vi "ALARM Catch Error.vi"(8 "error in (no error)":errorcluster, 9 "Data":variant, 10 "Message Queues out":T2, 11 "Hardware Resources in":T1={"LOG REF"=refnum, "Writer Queue"=refnum, "Log Path"=path "", "UPS standby"=FALSE, "status code"=5001, "SP"=[], "Over Sens Status"=[]}) -> (0 "error out":errorcluster, 3 "Hardware Resources out":T1={"LOG REF"=refnum, "Writer Queue"=refnum, "Log Path"=path "", "UPS standby"=FALSE, "status code"=5001, "SP"=[], "Over Sens Status"=[]})   [LabVIEW 2020, in "QCT ALARM.lvlib"]
uses:
  QCT ALARM.lvlib
  support/Message Queue/All Message Queues.ctl
  support/Message Queue/Message Cluster.ctl
  ALARM Configuration.ctl
  support/HW Message Cluster.ctl
  support/Message Queue/Enqueue Message (Single).vi
  support/Message Queue/Message Queue.lvlib
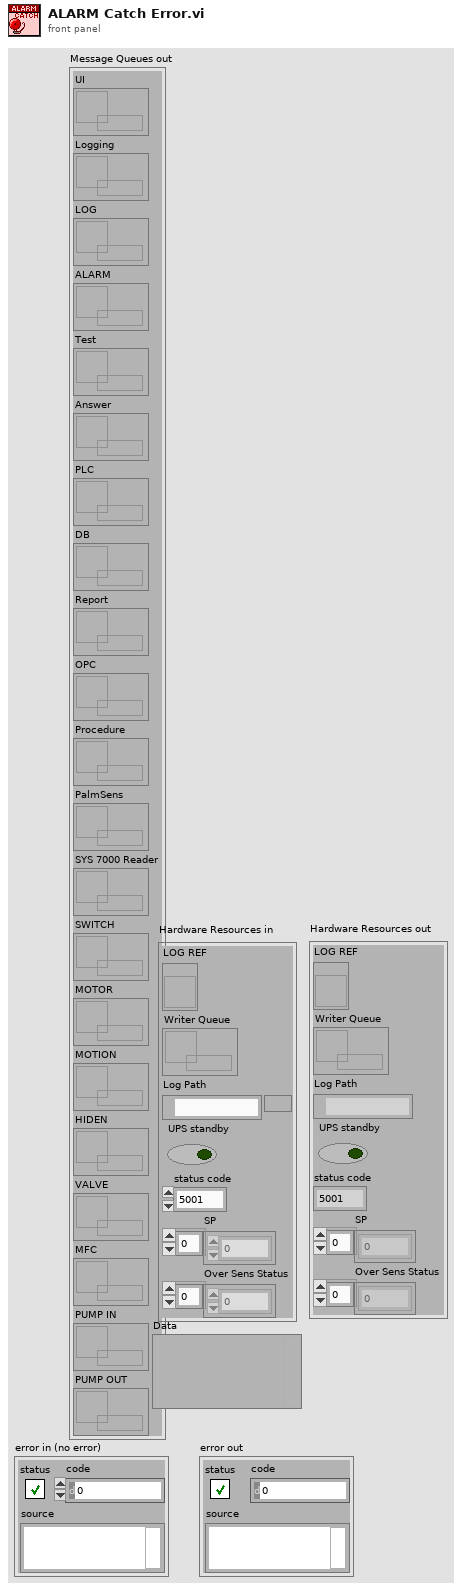
[diagram p1: front panel]
types:
  T1 = typedef "QCT ALARM.lvlib/ALARM Configuration.ctl" = cluster{"LOG REF":refnum<vi>, "Writer Queue":refnum<queue>, "Log Path":path, "UPS standby":bool, "status code":i32, "SP":dbl[], "Over Sens Status":dbl[]}
  T2 = typedef "Message Queue.lvlib/All Message Queues.ctl" = cluster{"UI":refnum<queue>, "Logging":refnum<queue>, "LOG":refnum<queue>, "ALARM":refnum<queue>, "Test":refnum<queue>, "Answer":refnum<queue>, "PLC":refnum<queue>, "DB":refnum<queue>, "Report":refnum<queue>, "OPC":refnum<queue>, "Procedure":refnum<queue>, "PalmSens":refnum<queue>, "SYS 7000 Reader":refnum<queue>, "SWITCH":refnum<queue>, "MOTOR":refnum<queue>, "MOTION":refnum<queue>, "HIDEN":refnum<queue>, "VALVE":refnum<queue>, "MFC":refnum<queue>, "PUMP IN":refnum<queue>, "PUMP OUT":refnum<queue>}
  T3 = typedef "Message Queue.lvlib/Message Cluster.ctl" = cluster{"Message":string, "Message Data":variant}
  T4 = typedef "Message Queue.lvlib/HW Message Cluster.ctl" = cluster{"Writer Queue":refnum<queue>, "Writer Data":T3}
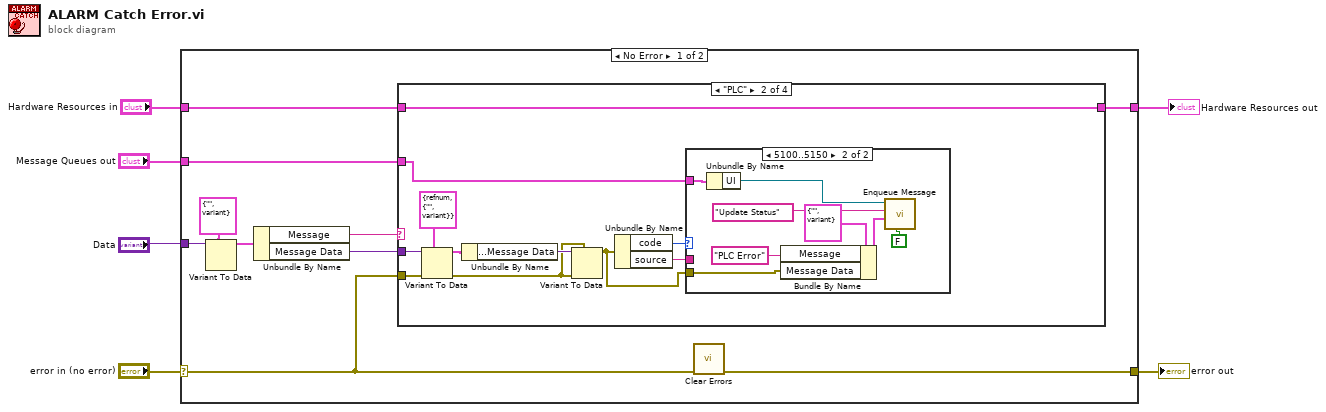
[diagram p0: block diagram]
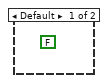
[diagram p3: hidden frame]
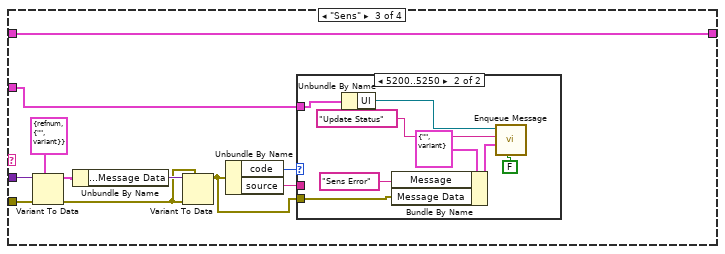
[diagram p4: hidden frame]
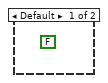
[diagram p5: hidden frame]
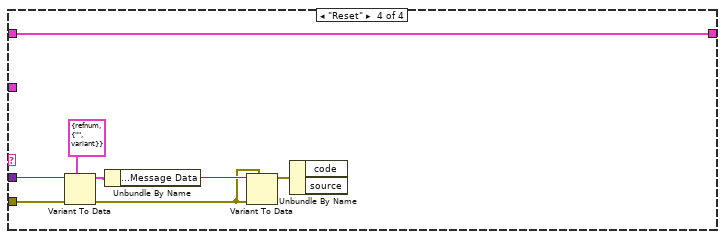
[diagram p6: hidden frame]
diagram:
  n1 = case shown="No Error" "error in (no error)" {
    selector: "error in (no error)" -> [w9 w65]
    tunnel: [w16 w65] -> w5
    tunnel: "Message Queues out" -> [w15 _]
    tunnel: "Data" -> [w14 _]
    tunnel: [w8 w64] -> w2
    tunnel: "Hardware Resources in" -> [w7 w64]
    frame No Error {
      n2 = Variant To Data(type=T3 {"Message"="", "Message Data"=variant} ("Message Cluster"), Variant=w14) -> (data=w13:T3)  [unwired: 1 in, 1 out]
      n3 = Unbundle By Name(w13) -> ("Message"=w11:string, "Message Data"=w10:variant)
      n4 = case shown="\"PLC\"" w11 {
        tunnel: w15 -> [_ w28 w47 _]
        tunnel: w10 -> [_ w25 w44 w61]
        tunnel: w9 -> [_ w23 w42 w59]
        tunnel: [w17 w19 w38 w56] -> w8
        tunnel: w7 -> [w17 w19 w38 w56]
        frame Default {
        }
        frame "PLC" {
          n5 = Variant To Data(error in=w23, type=T4 {"Writer Queue"=refnum, "Writer Data"={"Message"="", "Message Data"=variant}} ("HW Message"), Variant=w25) -> (data=w26:T4, error out=w22:errorcluster)
          n6 = Unbundle By Name(w26) -> ("Writer Data.Message Data"=w24:variant)
          n7 = Variant To Data(error in=w22, type=w22, Variant=w24) -> (data=w18:errorcluster)  [unwired: 1 out]
          n8 = Unbundle By Name(w18) -> ("code"=w21:i32, "source"=w20:string)
          n9 = case shown="5100..5150" w21 {
            tunnel: w20 -> [_ _]
            tunnel: w28 -> [_ w36]
            tunnel: w18 -> [_ w29]
            frame Default {
              (unwired) FALSE
            }
            frame 5100..5150 {
              n10 = Unbundle By Name(w36) -> ("UI"=w35:refnum<queue>)
              n11 = Bundle By Name(cluster=T3 {"Message"="", "Message Data"=variant} ("Message Cluster"), "Message"="PLC Error", "Message Data"=w29) -> (w31:T3)
              n12 = call-poly "Enqueue Message.vi"("Priority Message? (F)"=FALSE, "Message Data"=w31, "Message"="Update Status", "Message Queue"=w35) -> ()  [unwired: 6 in, 2 out]
            }
          }
        }
        frame "Sens" {
          n13 = Variant To Data(error in=w42, type=T4 {"Writer Queue"=refnum, "Writer Data"={"Message"="", "Message Data"=variant}} ("HW Message"), Variant=w44) -> (data=w45:T4, error out=w41:errorcluster)
          n14 = Unbundle By Name(w45) -> ("Writer Data.Message Data"=w43:variant)
          n15 = Variant To Data(error in=w41, type=w41, Variant=w43) -> (data=w37:errorcluster)  [unwired: 1 out]
          n16 = Unbundle By Name(w37) -> ("code"=w40:i32, "source"=w39:string)
          n17 = case shown="5200..5250" w40 {
            tunnel: w39 -> [_ _]
            tunnel: w47 -> [_ w55]
            tunnel: w37 -> [_ w48]
            frame Default {
              (unwired) FALSE
            }
            frame 5200..5250 {
              n18 = Unbundle By Name(w55) -> ("UI"=w54:refnum<queue>)
              n19 = Bundle By Name(cluster=T3 {"Message"="", "Message Data"=variant} ("Message Cluster"), "Message"="Sens Error", "Message Data"=w48) -> (w50:T3)
              n20 = call-poly "Enqueue Message.vi"("Priority Message? (F)"=FALSE, "Message Data"=w50, "Message"="Update Status", "Message Queue"=w54) -> ()  [unwired: 6 in, 2 out]
            }
          }
        }
        frame "Reset" {
          n21 = Variant To Data(error in=w59, type=T4 {"Writer Queue"=refnum, "Writer Data"={"Message"="", "Message Data"=variant}} ("HW Message"), Variant=w61) -> (data=w62:T4, error out=w58:errorcluster)
          n22 = Unbundle By Name(w62) -> ("Writer Data.Message Data"=w60:variant)
          n23 = Variant To Data(error in=w58, type=w58, Variant=w60) -> (data=w57:errorcluster)  [unwired: 1 out]
          n24 = Unbundle By Name(w57) -> ()  [unwired: 2 out]
        }
      }
      n25 = call <vilib>:"Clear Errors.vi"("error in (no error)"=w9) -> ("error out"=w16:errorcluster)  [unwired: 5 in, 1 out]
    }
    frame Error {
    }
  }
  "error out" <- w5
  "Hardware Resources out" <- w2
